vi "Guided Calibration Get Ports.vi"(8 "error in (no error)":errorcluster {"code" format="%.0x"}, 9 "ValBufferSize":i32=2048, 10 "ChannelNumber":i32 format="%.0g", 11 "instrument handle":refnum<k15>) -> (0 "error out":errorcluster {"code" format="%.0x"}, 1 "ValActualSize":i32, 2 "Val":i32[](array[numeric]), 3 "instrument handle out":refnum<k15>)   [LabVIEW 2014, in "Agilent NA.lvlib"]
doc: "Get ports to be calibrated for the given channel."
uses:
  Agilent NA.lvlib
  AgNA.dll
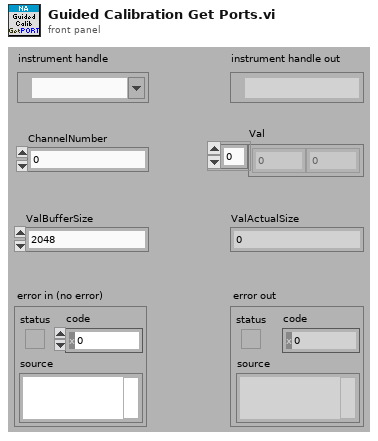
[diagram p1: front panel]
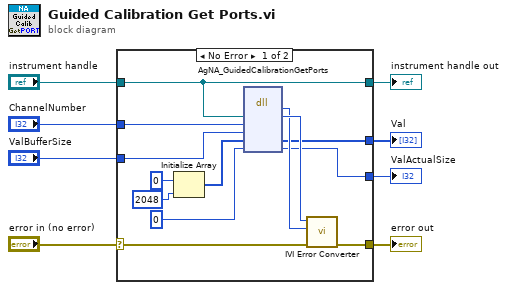
[diagram p0: block diagram]
diagram:
  n1 = case shown="No Error" "error in (no error)" {
    selector: "error in (no error)" -> [w19 w23]
    tunnel: [w18 w23] -> w8
    tunnel: "ChannelNumber" -> [w17 _]
    tunnel: "ValBufferSize" -> [w16 _]
    tunnel: [w12 _] -> w4
    tunnel: [w10 _] -> w3
    tunnel: [w9 w22] -> w2
    tunnel: "instrument handle" -> [w9 w22]
    frame No Error {
      n2 = Initialize Array(0 ("element"), 2048 ("dimension size")) -> (w15:i32[])
      n3 = dll-call lib="AgNA**.dll" fn="AgNA_GuidedCalibrationGetPorts"("Vi"=w9, "ChannelNumber"=w17, "ValBufferSize"=w16, "Val"=w15, "ValActualSize"=0) -> (w20:i32, "Vi"=w21:u32, "Val"=w12:i32[], "ValActualSize"=w10:i32)  [unwired: 5 in, 2 out]
      n4 = call "IVI Error Converter.vi"("error in (no error)"=w19, "IVI error code (0)"=w20, "instrument handle"=w21) -> ("error out"=w18:errorcluster)  [unwired: 7 in, 1 out]
    }
    frame Error {
    }
  }
  "error out" <- w8
  "instrument handle out" <- w2
  "Val" <- w4
  "ValActualSize" <- w3
